vi "Maxes.vi"(1 "Array":dbl[](array[numeric]), 2 "Number of max":i32) -> (0 "Values and Indx":dbl[][](array[numeric]))   [LabVIEW 2009]
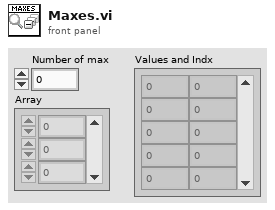
[diagram p1: front panel]
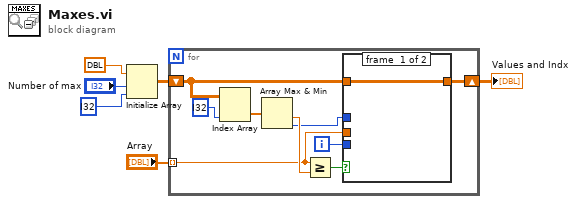
[diagram p0: block diagram]
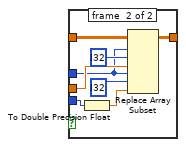
[diagram p2: hidden frame]
diagram:
  n1 = Initialize Array(dbl ?, "Number of max", i32 ? ("dimension size")) -> (w4:dbl[][])
  n2 = for {
    tunnel: "Array" -> [w7] mode=indexing
    shift-right: [w12] -> w1
    shift-left: w4 -> [w13]
    i -> [w8]
    n3 = Index Array(array=w13, index (col)=i32 ? ("disabled index (col)")) -> (element=w14:dbl[])  [unwired: 1 in]
    n4 = Array Max & Min(array=w14) -> (min value=w11:dbl, min index (indices)=w10:i32)  [unwired: 2 out]
    n5 = Greater Or Equal?(x=w7, y=w11) -> (x >= y?=w9:bool)
    n6 = case shown="True" w9 {
      tunnel: w13 -> [w16 w23]
      tunnel: [w16 w24] -> w12
      tunnel: w7 -> [_ w21]
      tunnel: w8 -> [_ w18]
      tunnel: w10 -> [_ w20]
      frame #0 {
      }
      frame #1 {
        n7 = To Double Precision Float(number=w18) -> (double precision float=w17:dbl)
        n8 = Replace Array Subset(array=w23, new element #1=w21, index (row) #1=w20, index (col) #1=i32 ? ("disabled index (col)"), new element #2=w17, index (row) #2=w20, index (col) #2=i32 ? ("disabled index (col)")) -> (w24:dbl[][])
      }
    }
  }
  "Values and Indx" <- w1
